vi "Wait Socket (TCP).vi"(8 "error in (no error)":errorcluster, 9 "timeout ms (25000)":u32=25000, 10 "tcp connection":refnum<k5>, 11 "session":T1) -> (0 "error out":errorcluster)   [LabVIEW 2017, in "libssh2.lvlib"]
doc: "Wait for data on a TCP connection in reading or writing direction as indicated by the session."
uses:
  libssh2.lvlib
  Session Refnum.ctl
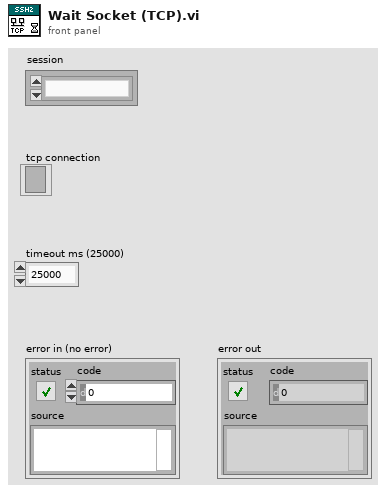
[diagram p1: front panel]
types:
  T1 = typedef "libssh2.lvlib/Session Refnum.ctl" = refnum<k1>
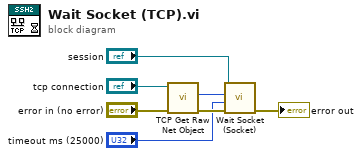
[diagram p0: block diagram]
diagram:
  n1 = call <vilib>:"TCP Get Raw Net Object.vi"("error in (no error)"="error in (no error)", "connection ID"="tcp connection") -> ("error out"=w4:errorcluster, "raw net object"=w1:u64)  [unwired: 7 in, 1 out]
  n2 = call "Wait Socket (Socket).vi"("error in (no error)"=w4, "timeout ms (25000)"="timeout ms (25000)", "socket"=w1, "session"="session") -> ("error out"=→"error out":errorcluster)  [unwired: 7 in]
